vi "write_to_serial.vi"(9 "value in":T1, 10 "address in":i16, 11 "VISA Refnum in":refnum<visa-resource-name>) -> ()   [LabVIEW 2015]
uses:
  Control 1.ctl
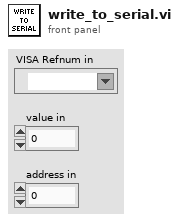
[diagram p1: front panel]
types:
  T1 = typedef "Control 1.ctl" = dbl
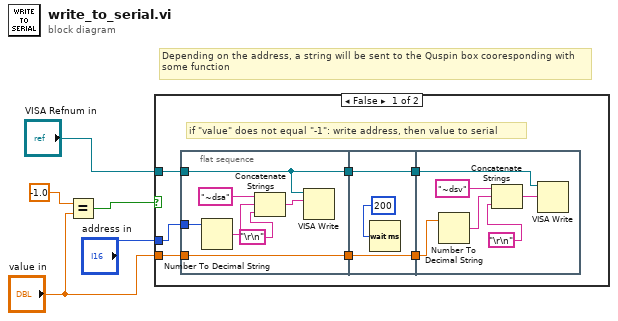
[diagram p0: block diagram]
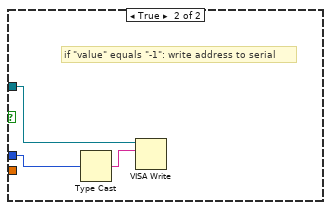
[diagram p2: hidden frame]
diagram:
  # "Depending on the address, a string will be sent to the Quspin box cooresponding with some function"
  n1 = Equal?(x=T1 -1.0, y="value in") -> (x = y?=w2:bool)
  n2 = case shown="False" w2 {
    tunnel: "address in" -> [w8 w29]
    tunnel: "value in" -> [w7 _]
    tunnel: "VISA Refnum in" -> [w6 w31]
    frame False {
      # "if \"value\" does not equal \"-1\": write address, then value to serial"
      n3 = flat-sequence {
        tunnel: [w14] -> w12
        tunnel: w8 -> [w17]
        tunnel: w7 -> [w15]
        tunnel: [w15] -> w11
        tunnel: w6 -> [w14]
        tunnel: w12 -> [w21]
        tunnel: [w21] -> w10
        tunnel: w11 -> [w20]
        tunnel: [w20] -> w9
        tunnel: w10 -> [w24]
        tunnel: w9 -> [w25]
        frame #0 {
          n4 = Number To Decimal String(number=w17) -> (decimal integer string=w16:string)  [unwired: 1 in]
          n5 = Concatenate Strings("~dsa" ("string"), w16, "\r\n") -> (w18:string)
          n6 = VISA Write(VISA resource name=w14, write buffer=w18) -> ()  [unwired: 1 in, 3 out]
        }
        frame #1 {
          n7 = Wait (ms)(milliseconds to wait=u32 200) -> ()  [unwired: 1 out]
        }
        frame #2 {
          n8 = Number To Decimal String(number=w25) -> (decimal integer string=w26:string)  [unwired: 1 in]
          n9 = Concatenate Strings("~dsv" ("string"), w26, "\r\n") -> (w27:string)
          n10 = VISA Write(VISA resource name=w24, write buffer=w27) -> ()  [unwired: 1 in, 3 out]
        }
      }
    }
    frame True {
      # "if \"value\" equals \"-1\": write address to serial"
      n11 = Type Cast(x=w29) -> (*(type *) &x=w30:string)  [unwired: 1 in]
      n12 = VISA Write(VISA resource name=w31, write buffer=w30) -> ()  [unwired: 1 in, 3 out]
    }
  }
